vi "ExSubInitCamera.vi"(2 "error in (no error)":errorcluster, 3 "Focus / Acquire Mode":u32=1 min=1 max=5 step=1, 4 "Camera Handle":u32) -> (0 "error out":errorcluster, 1 "Camera Handle":u32)   [LabVIEW 2010]
uses:
  GlobalAcquireFocusFlag.vi
  GlobalExposure.vi
  GlobalFramesToStr.vi
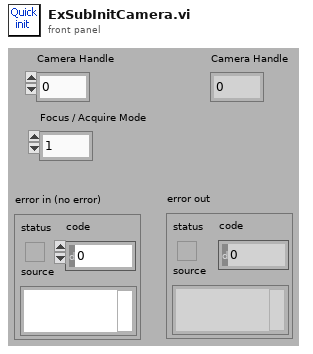
[diagram p1: front panel]
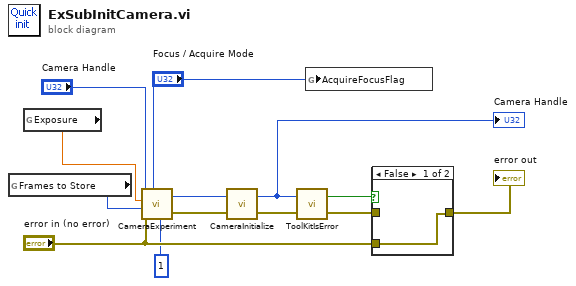
[diagram p0: block diagram]
diagram:
  n1 = global read "GlobalFramesToStr.vi" "Frames to Store"() -> (w9:u32)
  n2 = global read "GlobalExposure.vi" "Exposure"() -> (w10:dbl)
  n3 = call <userlib>:"CameraExperiment.vi"("Number of Accumulations"=1, "Acquire / Focus Flag"="Focus / Acquire Mode", "error in"="error in (no error)", "Number of Images"=w9, "Exposure (sec)"=w10, "Camera Handle"="Camera Handle") -> ("error out"=w8:errorcluster, "Camera Handle"=w7:u32)
  n4 = call <userlib>:"CameraInitialize.vi"("error in"=w8, "Camera Handle"=w7) -> ("error out"=w6:errorcluster, "Camera Handle"=w5:u32)
  "Camera Handle" <- w5
  n5 = call <userlib>:"ToolKitIsError.vi"("error in"=w6, "Reserved"=w5) -> ("error out"=w12:errorcluster, "Error Flag"=w13:bool)
  n6 = global write "GlobalAcquireFocusFlag.vi" "AcquireFocusFlag"("Focus / Acquire Mode") -> ()
  n7 = case shown="False" w13 {
    tunnel: w12 -> [_ w15]
    tunnel: [w14 w15] -> w4
    tunnel: "error in (no error)" -> [w14 _]
    frame False {
    }
    frame True {
    }
  }
  "error out" <- w4
